vi "Query Numeric (Harmonics).vi"(8 "error in (no error)":errorcluster, 10 "Item (1)":i32=1 min=1 max=64 step=1, 11 "VISA resource name":refnum<visa-resource-name>) -> (0 "error out":errorcluster, 2 "Function":string, 3 "VISA resource name out":refnum<visa-resource-name>)   [LabVIEW 2021, in "Yokogawa WT1800 Series.lvlib"]
doc: "Queries the output item (function and element) of the specified harmonic measurement\nnumeric list data item."
uses:
  <instrlib>/Yokogawa WT1800 Series/Yokogawa WT1800 Series.lvlib
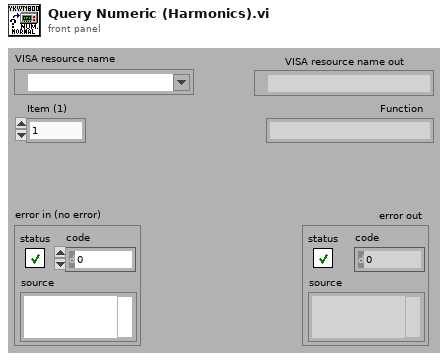
[diagram p1: front panel]
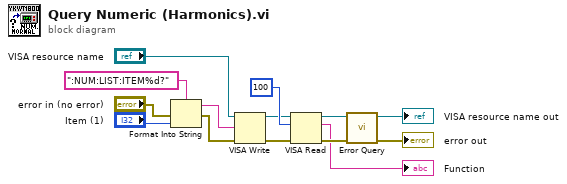
[diagram p0: block diagram]
diagram:
  n1 = Format Into String(format string=":NUM:LIST:ITEM%d?" ("形式文字列"), error in="error in (no error)", "Item (1)") -> (resulting string=w7:string, error out=w8:errorcluster)  [unwired: 1 in]
  n2 = VISA Write ("VISA書き込み")(VISA resource name="VISA resource name", write buffer=w7, error in (no error)=w8) -> (VISA resource name out=w5:refnum<visa-resource-name>, error out=w3:errorcluster)  [unwired: 1 out]
  n3 = VISA Read ("VISA読み取り")(VISA resource name=w5, byte count=u32 100, error in (no error)=w3) -> (VISA resource name out=w4:refnum<visa-resource-name>, read buffer=→"Function":string, error out=w2:errorcluster)  [unwired: 1 out]
  n4 = call <instrlib>:"Error Query.vi"("error in (no error)"=w2, "VISA resource name"=w4) -> ("error out"=→"error out":errorcluster, "VISA resource name out"=→"VISA resource name out":refnum<visa-resource-name>)  [unwired: 6 in, 2 out]
